vi "Load ROI file.vi"(11 "Experiment data folder path":path) -> (1 "Number of ROI":i32, 2 "ROI Data (header removed)":dbl[][](array[numeric]), 3 "ROI columns header":string[](array[string]), 5 "Version index (-1 = latest version)":i32)   [LabVIEW 2013]
uses:
  Typedefs/Enum-Which file or folder.ctl
  Program Files (x86)/National Instruments/LabVIEW 2013/user.lib/My Palettes.lib/Files & paths/Spreadsheet/Read From Spreadsheet File (string)-Mod.vi
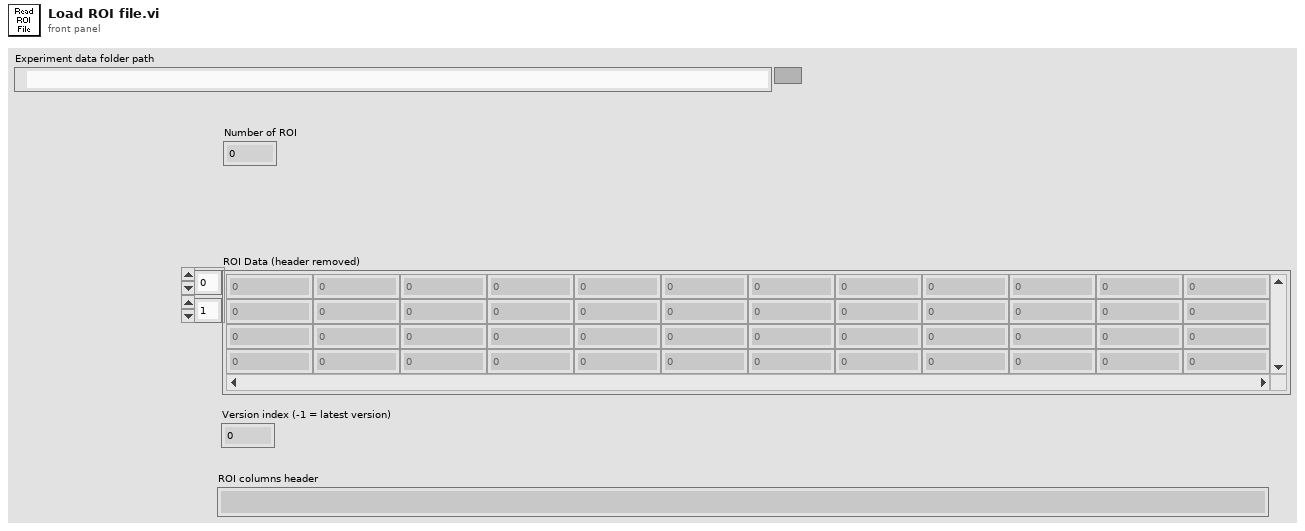
[diagram p1: front panel]
types:
  T1 = typedef "Enum-Which file or folder.ctl" = enum16{"ROI file", "Normalised ROI file", "Zplane Pockels values file", "Functional data folder"}
  T2 = typedef "Fixed strings.ctl" = cluster{"ROI file name":string, "Normalised ROI file name":string, "Zplane Pockels values file name":string, "Functional data folder name":string, "Experiment Header file name":string, "Z-stack images folder name":string, "Groups setup rel. path":string, "Groups text file rel. path":string, "TDMS files folder name (F.img)":string, "TDMS files folder name (V.acq)":string, "TDMS files folder name (Pl.acq)":string, "Cycle rel times sequence file":string, "Dynamically called VIs folder name":string, "Time Series folder base name":string}
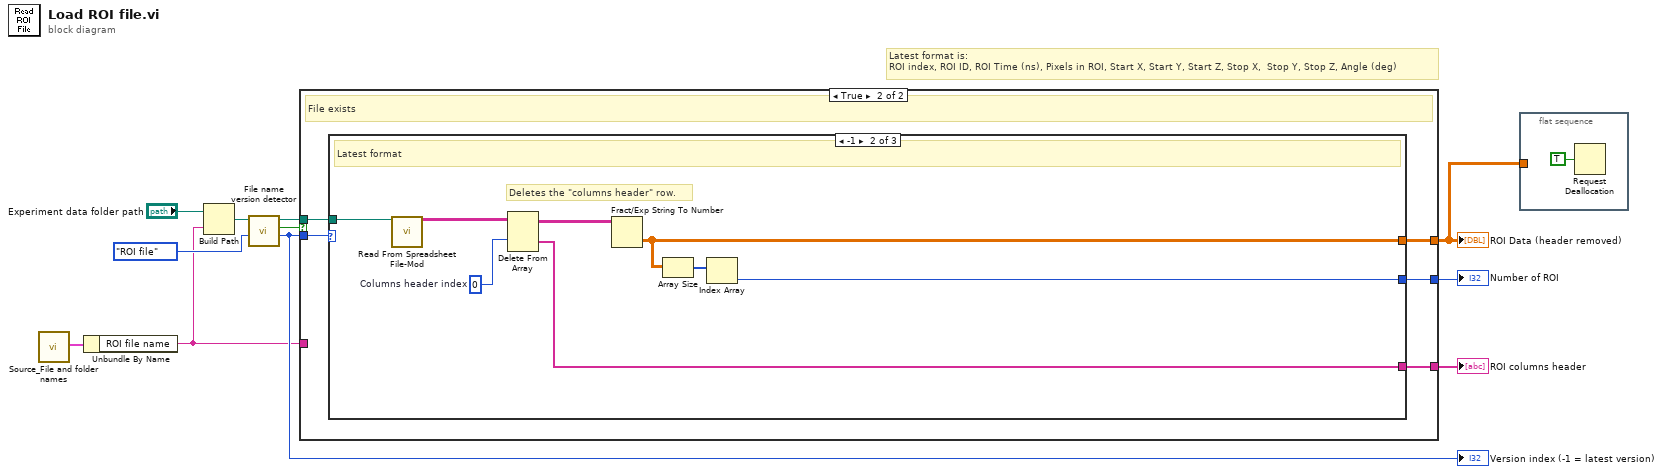
[diagram p0: block diagram]
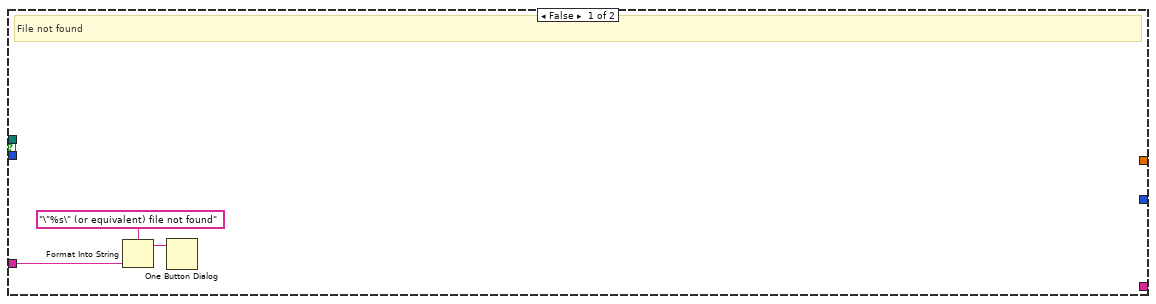
[diagram p2: hidden frame]
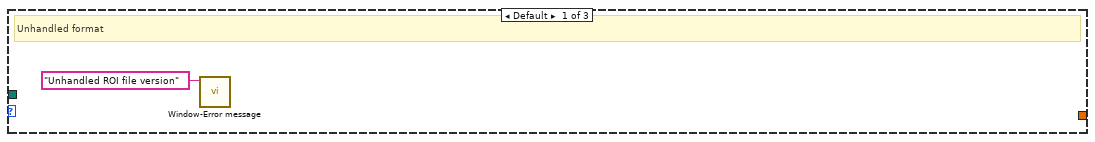
[diagram p3: hidden frame]
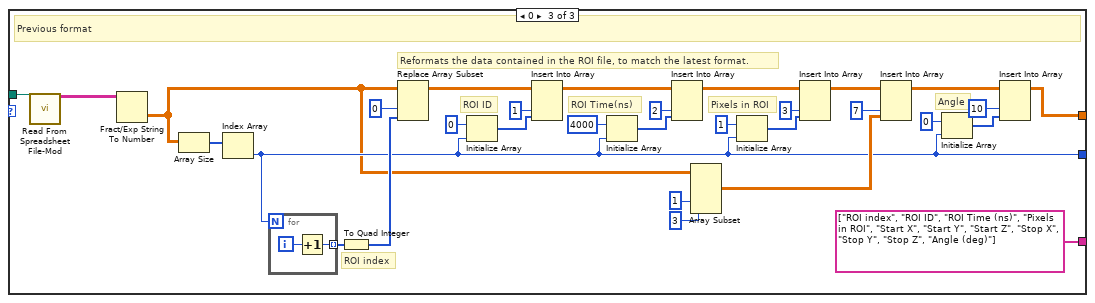
[diagram p4: hidden frame]
diagram:
  # "Latest format is:\nROI index,\tROI ID,\tROI Time (ns),\tPixels in ROI,\tStart X,\tStart Y,\tStart Z,\tStop X,\t Stop Y,\tStop Z,\tAngle (deg)"
  n1 = call "Source_File and folder names.vi"() -> ("Fixed strings"=w2:T2)  [unwired: 1 in]
  n2 = Unbundle By Name(w2) -> ("ROI file name"=w3:string)
  n3 = Build Path(base path="Experiment data folder path", name or relative path=w3) -> (appended path=w9:path)
  n4 = call "File name version detector.vi"("Which file/folder?"=Enum-Which_file_or_folder."ROI file", "Path in"=w9) -> ("Version index (-1 = latest version)"=w7:i32, "file or folder exists"=w6:bool, "Path out"=w8:path)  [unwired: 7 in]
  "Version index (-1 = latest version)" <- w7
  n5 = case shown="True" w6 {
    tunnel: [_ w19] -> w1
    tunnel: [_ w18] -> w10
    tunnel: w8 -> [_ w17]
    tunnel: w7 -> [_ w16]
    tunnel: [_ w15] -> w5
    tunnel: w3 -> [w12 _]
    frame False {
      # "File not found"
      n6 = Format Into String(format string="\"%s\" (or equivalent) file not found" ("message"), w12) -> (resulting string=w13:string)  [unwired: 2 in, 1 out]
      n7 = One Button Dialog(message=w13) -> ()  [unwired: 1 in, 1 out]
    }
    frame True {
      # "File exists"
      n8 = case shown="-1" w16 {
        tunnel: [_ w25 w31] -> w19
        tunnel: [_ w24 w32] -> w18
        tunnel: w17 -> [_ w21 w58]
        tunnel: [_ w23 string[] ["ROI index", "ROI ID", "ROI Time (ns)", "Pixels in ROI", "Start X", "Start Y", "Start Z", "Stop X", "Stop Y", "Stop Z", "Angle (deg)"] ("all rows")] -> w15
        frame Default {
          # "Unhandled format"
          n9 = call "Window-Error message.vi"("Message"="Unhandled ROI file version" ("message")) -> ()  [unwired: 10 in, 1 out]
        }
        frame -1 {
          w27 = 0  # Columns header index
          # "Deletes the \"columns header\" row."
          # "Latest format"
          n10 = call-poly "Read From Spreadsheet File-Mod.vi"("file path (dialog if empty)"=w21) -> ("all rows"=w22:string[][])  [unwired: 9 in, 5 out]
          n11 = Delete From Array(array=w22, index (row)=w27) -> (deleted portion=w23:string[], array with subset deleted=w28:string[][])  [unwired: 2 in]
          n12 = Fract/Exp String To Number(string=w28) -> (number=w25:dbl[][])  [unwired: 3 in, 1 out]
          n13 = Array Size(array=w25) -> (size(s)=w26:i32[])
          n14 = Index Array(array=w26) -> (element=w24:i32)  [unwired: 1 in]
        }
        frame 0 {
          # "Reformats the data contained in the ROI file, to match the latest format."
          # "Pixels in ROI"
          # "Angle"
          # "ROI Time(ns)"
          # "ROI ID"
          # "ROI index"
          # "Previous format"
          n15 = call-poly "Read From Spreadsheet File-Mod.vi"("file path (dialog if empty)"=w58) -> ("all rows"=w29:string[][])  [unwired: 9 in, 5 out]
          n16 = Fract/Exp String To Number(string=w29) -> (number=w30:dbl[][])  [unwired: 3 in, 1 out]
          n17 = Array Size(array=w30) -> (size(s)=w59:i32[])
          n18 = Index Array(array=w59) -> (element=w32:i32)  [unwired: 1 in]
          n19 = for {
            N: w32 -> [_]
            tunnel: [w60] -> w55 mode=indexing
            i -> [w61]
            n20 = Increment(x=w61) -> (x+1=w60:i32)
          }
          n21 = To Quad Integer(1:w55) -> (0:w54:i64[])
          n22 = Replace Array Subset(array=w30, new element=w54, index (col)=0 ("disabled index (col)")) -> (w52:dbl[][])  [unwired: 1 in]
          n23 = Initialize Array(i64 0 ("element"), w32) -> (w51:i64[])
          n24 = Insert Into Array(array=w52, index (col)=1 ("disabled index (col)"), new element=w51) -> (w46:dbl[][])  [unwired: 1 in]
          n25 = Initialize Array(i64 4000 ("element"), w32) -> (w48:i64[])
          n26 = Insert Into Array(array=w46, index (col)=2 ("disabled index (col)"), new element=w48) -> (w34:dbl[][])  [unwired: 1 in]
          n27 = Array Subset(array=w30, index (col)=1 ("index (row)"), length (col)=3 ("length")) -> (w42:dbl[][])  [unwired: 2 in]
          n28 = Initialize Array(i64 1 ("element"), w32) -> (w36:i64[])
          n29 = Insert Into Array(array=w34, index (col)=3 ("disabled index (col)"), new element=w36) -> (w33:dbl[][])  [unwired: 1 in]
          n30 = Insert Into Array(array=w33, index (col)=7 ("disabled index (col)"), new element=w42) -> (w40:dbl[][])  [unwired: 1 in]
          n31 = Initialize Array(i64 0 ("element"), w32) -> (w39:i64[])
          n32 = Insert Into Array(array=w40, index (col)=10 ("disabled index (col)"), new element=w39) -> (w31:dbl[][])  [unwired: 1 in]
        }
      }
    }
  }
  "ROI Data (header removed)" <- w1
  "Number of ROI" <- w10
  "ROI columns header" <- w5
  n33 = flat-sequence {
    tunnel: w1 -> [_]
    frame #0 {
      n34 = Request Deallocation(TRUE ("flag")) -> ()
    }
  }
